vi "TCP IP Parse CoagMode.vi"(11 "JSON in":string) -> (2 "Value":T1, 3 "JSON out":string)   [LabVIEW 2015]
uses:
  Controls/Control_Fornax Mono1 Coag Enum.ctl
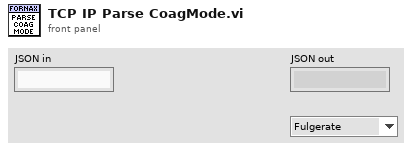
[diagram p1: front panel]
types:
  T1 = typedef "Control_Fornax Mono1 Coag Enum.ctl" = enum16{"Fulgerate", "Spray"}
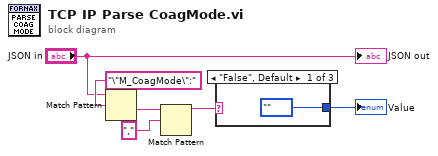
[diagram p0: block diagram]
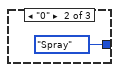
[diagram p2: hidden frame]
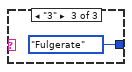
[diagram p3: hidden frame]
diagram:
  n1 = Match Pattern(string="JSON in", regular expression="\"M_CoagMode\":") -> (after substring=w4:string)  [unwired: 1 in, 3 out]
  n2 = Match Pattern(string=w4, regular expression=",") -> (before substring=w6:string)  [unwired: 1 in, 3 out]
  n3 = case shown="\"False\", Default" w6 {
    tunnel: [enum16{""}."" Control_Fornax_Mono1_Coag_Enum."Spray" ("Value") Control_Fornax_Mono1_Coag_Enum."Fulgerate" ("Value")] -> w1
    frame "False", Default {
    }
    frame "0" {
    }
    frame "3" {
    }
  }
  "Value" <- w1
  "JSON out" <- "JSON in"
